vi "Global Analog.vi"() -> ()   [LabVIEW 2026]
doc: "A global variable which contains setup information for analog systems.\n\nValid for Analog systems (but must be present for all other systems, too)."
panel:
  in  "Analog System":T1(array[cluster]) {"Conversion offset" format="%.2f"; "AO.MaxRate" format="%.2f"; "Gain (V)" format="%.7f"; "Offset (V)" format="%.7f"; "AI Sample Rate" format="%.2f"; "Upper voltage limit (V)" format="%.6f"; "Lower voltage limit (V)" format="%.6f"; "Velocity" format="%.2f"; "Conversion factor" format="%.2f"}
  # "Global Analog is a global variable which contains setup information for analog control."
  # "GKo, 24/10/07"
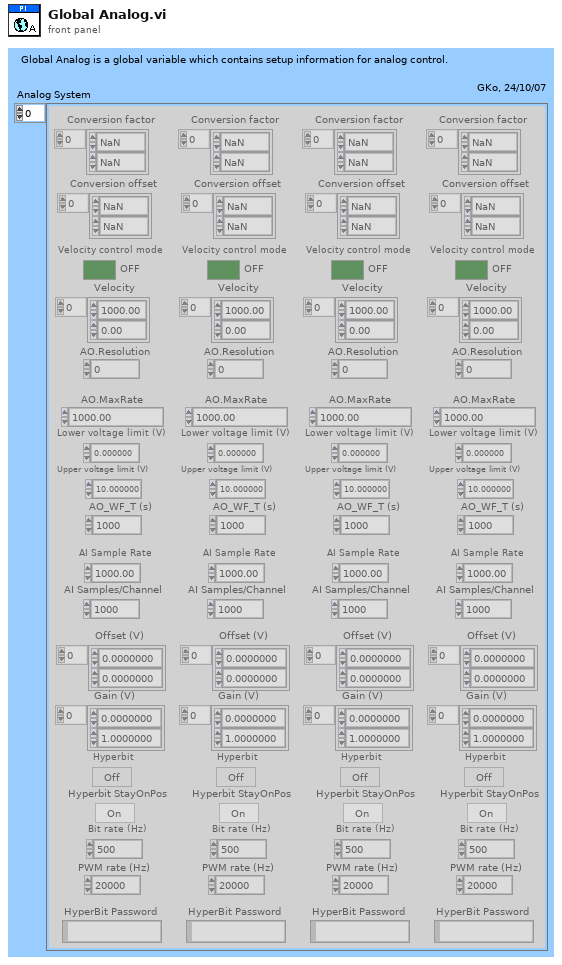
[diagram p1: front panel]
types:
  T1 = cluster{"Conversion factor":dbl[], "Velocity":dbl[], "Velocity control mode":bool, "AO.Resolution":dbl, "Lower voltage limit (V)":dbl, "Upper voltage limit (V)":dbl, "AO_WF_T (s)":dbl, "AI Sample Rate":dbl, "AI Samples/Channel":i32, "Hyperbit":bool, "Offset (V)":dbl[], "Hyperbit StayOnPos":bool, "Gain (V)":dbl[], "Bit rate (Hz)":dbl, "PWM rate (Hz)":dbl, "HyperBit Password":string, "AO.MaxRate":dbl, "Conversion offset":dbl[]}[]
diagram:
